vi "Actor Core.vi"(8 "error in":errorcluster, 11 "Measure Object in":refnum<class "Fluke Recorder.lvclass">) -> (0 "error out":errorcluster, 3 "Actor out":refnum<class "Actor.lvclass">)   [LabVIEW 2019, in "Fluke Recorder.lvclass"]
doc: "(<B>Filename</B>: Actor Framework.lvlib:Actor.lvclass:Actor Core.vi)\n\nReceives messages to the actor, reacts to them, and initiates any error handling that may shut the actor down.\n\nDescendant classes may override this VI to append parallel tasks for the actor to complete while it handles messages. Overrides use the Call Parent Method node."
uses:
  Fluke Recorder.lvclass
  <vilib>/ActorFramework/Actor/Actor.lvclass
  NHMFL_Core/Libraries/Instruments/Fluke/Fluke Configuration.ctl
  Instrument Actor/Instrument Actor.lvclass
panel:
  in  "Configuration":T1={"Channels"="201:203"}
  out "Name":string
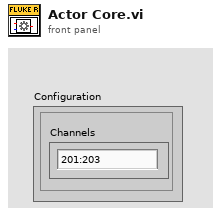
[diagram p1: front panel]
types:
  T1 = typedef "Fluke Configuration.ctl" = cluster{"Channels":string}
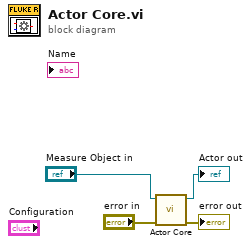
[diagram p0: block diagram]
diagram:
  n1 = call-parent "Actor Core.vi"("error in"="error in", "Measure Object in"="Measure Object in") -> ("error out"=→"error out":errorcluster, "Actor out"=→"Actor out":refnum<class "Actor.lvclass">)  [unwired: 8 in]
